vi "Overspeed Check.vi"(7 "reset(F)":bool, 8 "计时时长(ms)":u32=5000, 9 "reset value":bool, 11 "Signal":bool) -> (0 "变化过去时间(ms)":u32, 3 "signal(safe)":bool)   [LabVIEW 2017, in "Communicable State Machine.lvlib"]
uses:
  Communicable State Machine.lvlib
  f775c943-ffbb-439c-97f3-d96e010d4a15.vi
  2ae720ed-5104-4348-9eb6-9a272da77c80.vi
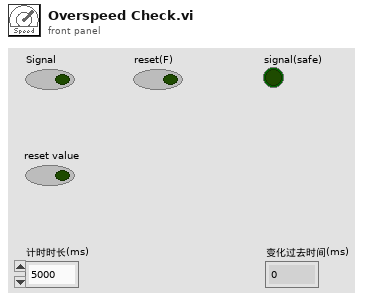
[diagram p1: front panel]
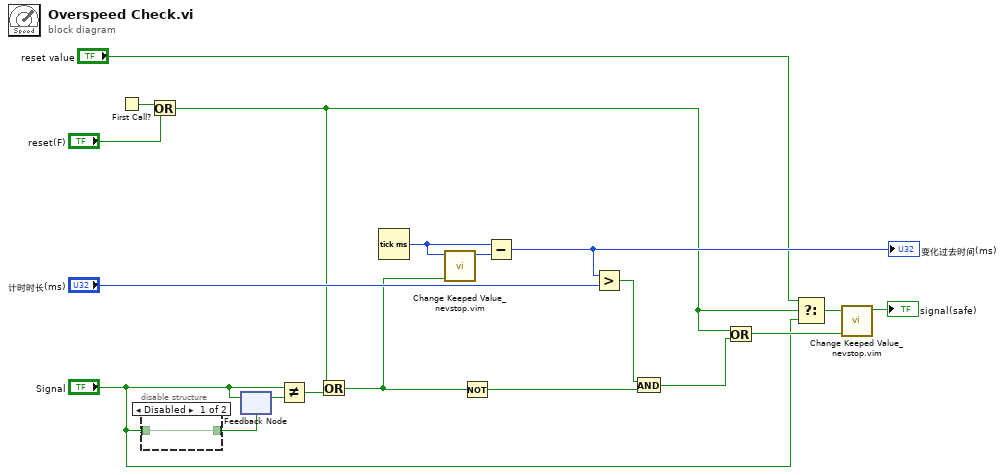
[diagram p0: block diagram]
diagram:
  n1 = First Call?() -> (First Call?: T/F=w19:bool)
  n2 = disable-structure shown="Disabled" {
    disable-tunnel: [w20 _] -> w3
    disable-tunnel: "Signal" -> [w20 _]
    frame Disabled {
    }
    frame Enabled {
    }
  }
  n3 = Or(x=w19, y="reset(F)") -> (x .or. y?=w5:bool)
  n4 = feedback #1(w3) -> (w4:bool)
  n5 = feedback-in #1("Signal") -> ()
  n6 = Not Equal?(x="Signal", y=w4) -> (x != y?=w1:bool)
  n7 = Or(x=w5, y=w1) -> (x .or. y?=w9:bool)
  n8 = Tick Count (ms)() -> (millisecond timer value=w11:u32)
  n9 = call "Change Keeped Value_nevstop.vim"("change?"=w9, "new value"=w11) -> ("keeped value"=w10:u32)  [unwired: 9 in]
  n10 = Not(x=w9) -> (.not. x?=w14:bool)
  n11 = Subtract(x=w11, y=w10) -> (x-y=w17:u32)
  "变化过去时间(ms)" <- w17
  n12 = Greater?(x=w17, y="计时时长(ms)") -> (0:w15:bool)
  n13 = And(x=w15, y=w14) -> (x .and. y?=w13:bool)
  n14 = Or(x=w5, y=w13) -> (x .or. y?=w8:bool)
  n15 = Select(t="reset value", s=w5, f="Signal") -> (s? t:f=w7:bool)
  n16 = call "Change Keeped Value_nevstop.vim"("change?"=w8, "new value"=w7) -> ("keeped value"=→"signal(safe)":bool)  [unwired: 9 in]
